vi "WPI_SimpleGyroFGV.vi"(7 "Operation":enum16{"set", "get"}(ring), 8 "Rate":dbl, 9 "Angle":dbl, 10 "Reset":bool, 11 "SimpleGyroDevRef":T1) -> (0 "Rate":dbl, 1 "Angle":dbl, 2 "Reset?":bool, 3 "SimpleGyroDevRef":T1)   [LabVIEW 2015, in "SimpleGyro.lvlib"]
uses:
  SimpleGyro.lvlib
  WPI_SimpleGyroDevRef.ctl
  <vilib>/Rock Robotics/SystemInterfaces/spilib/spi_bus.ctl
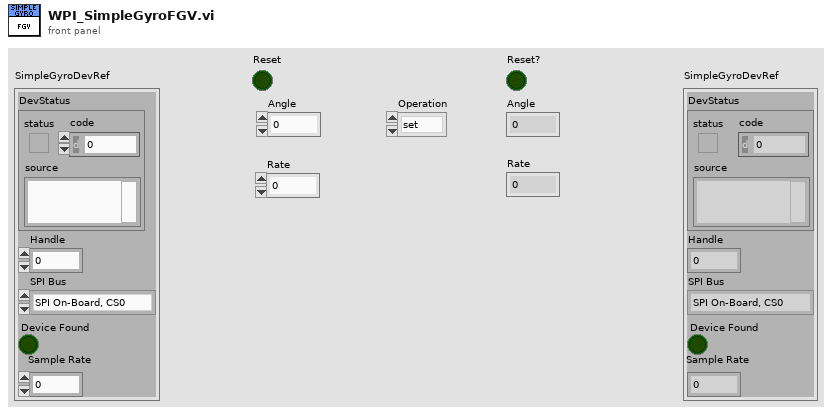
[diagram p1: front panel]
types:
  T1 = typedef "SimpleGyro.lvlib/WPI_SimpleGyroDevRef.ctl" = cluster{"DevStatus":errorcluster, "Handle":i32, "SPI Bus":T2, "Device Found":bool, "Sample Rate":dbl}
  T2 = typedef "spi_bus.ctl" = enum16{"SPI On-Board, CS0", "SPI On-Board, CS1", "SPI On-Board, CS2", "SPI On-Board, CS3", "SPI MXP", "Invalid"}
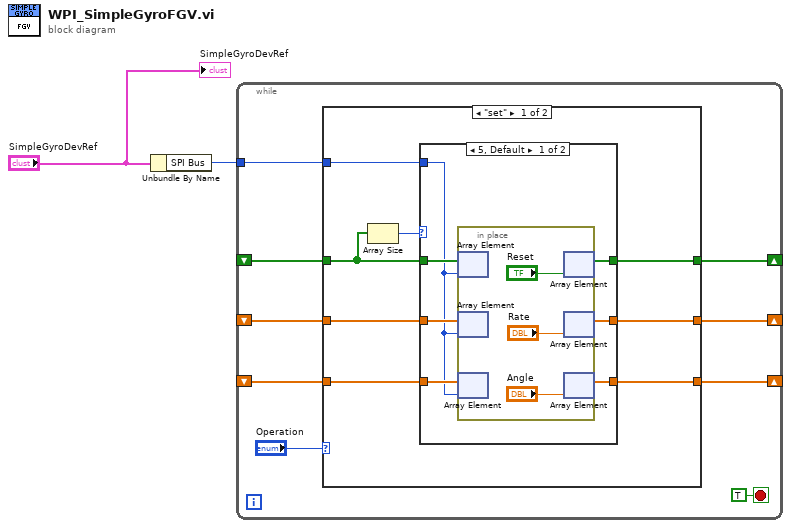
[diagram p0: block diagram]
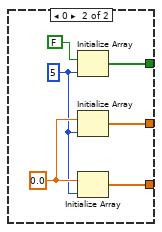
[diagram p2: hidden frame]
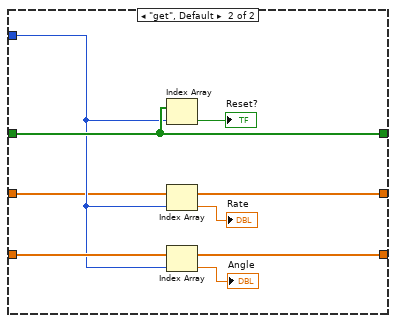
[diagram p3: hidden frame]
diagram:
  n1 = Unbundle By Name("SimpleGyroDevRef") -> ("SPI Bus"=w2:T2)
  n2 = while {
    tunnel: w2 -> [w5]
    shift-right: [w9] -> _
    shift-left: _ -> [w7]
    shift-right: [w8] -> _
    shift-left: _ -> [w6]
    shift-right: [w4] -> _
    shift-left: _ -> [w3]
    stop <- TRUE stop-if-true
    n3 = case shown="\"set\"" "Operation" {
      tunnel: [w19 w42] -> w9
      tunnel: [w18 w41] -> w8
      tunnel: w7 -> [w16 w42]
      tunnel: w6 -> [w15 w41]
      tunnel: w5 -> [w14 w38]
      tunnel: [w13 w37] -> w4
      tunnel: w3 -> [w12 w37]
      frame "set" {
        n4 = Array Size(array=w16) -> (size(s)=w17:i32)
        n5 = case shown="5, Default" w17 {
          tunnel: [w24 w34] -> w19
          tunnel: [w23 w33] -> w18
          tunnel: w16 -> [w26 _]
          tunnel: w15 -> [w25 _]
          tunnel: w14 -> [w21 _]
          tunnel: [w20 w32] -> w13
          tunnel: w12 -> [w22 _]
          frame 5, Default {
            n6 = in-place {
              n7 = in-place-array #1(w26, w21) -> ()  [unwired: 1 out]
              n8 = in-place-array #2(w22, w21) -> ()  [unwired: 1 out]
              n9 = in-place-array #3(w25, w21) -> ()  [unwired: 1 out]
              n10 = in-place-array #1("Reset") -> (w24:bool[])  [unwired: 1 out]
              n11 = in-place-array #2("Rate") -> (w20:dbl[])  [unwired: 1 out]
              n12 = in-place-array #3("Angle") -> (w23:dbl[])  [unwired: 1 out]
            }
          }
          frame 0 {
            w31 = 0.0 ("Angle")
            w30 = 5 ("dimension size")
            n13 = Initialize Array(FALSE ("Reset"), w30) -> (w34:bool[])
            n14 = Initialize Array(w31, w30) -> (w32:dbl[])
            n15 = Initialize Array(w31, w30) -> (w33:dbl[])
          }
        }
      }
      frame "get", Default {
        n16 = Index Array(array=w42, index=w38) -> (element=→"Reset?":bool)
        n17 = Index Array(array=w37, index=w38) -> (element=→"Rate":dbl)
        n18 = Index Array(array=w41, index=w38) -> (element=→"Angle":dbl)
      }
    }
  }
  "SimpleGyroDevRef" <- "SimpleGyroDevRef"
